vi "SequenceNodeUI.vi"() -> ()   [LabVIEW 2015, in "CleanupCategoryNode.lvclass"]
doc: "Copyright 2017 National Instruments Corporation\n\nLicensed under the Apache License, Version 2.0 (the \"License\"); you may not use this file except in compliance with the License. You may obtain a copy of the License at http://www.apache.org/licenses/LICENSE-2.0\nUnless required by applicable law or agreed to in writing, software distributed under the License is distributed on an \"AS IS\" BASIS, WITHOUT WARRANTIES OR CONDITIONS OF ANY KIND, either express or implied. See the License for the specific language governing permissions and limitations under the License."
uses:
  CleanupCategoryNode.lvclass
  <vilib>/NI/Configuration Framework/Node/NodeRef.ctl
  <vilib>/NI/Configuration Framework/Node/NISE_CEF_Node.lvclass
  <vilib>/NI/AMC/Message Queue.ctl
  <vilib>/NI/AMC/Message.ctl
  <vilib>/NI/Tools/Keyed Array/KeyedArray.ctl
  <vilib>/NI/Configuration Framework/Node/UserEventRef.ctl
  <vilib>/NI/Configuration Framework/Controls/EventCluster.ctl
  <vilib>/NI/AMC/Create Single Message.vi
  <vilib>/NI/AMC/Update Message Routing Info.vi
  <vilib>/NI/AMC/Send Message.vi
  <vilib>/NI/AMC/AMC.lvlib
  <vilib>/NI/Tools/Keyed Array/Tools_KeyedArray.lvlib
  <vilib>/NI/Configuration Framework/NISE_CEF_TreeControl.lvlib
panel:
  in  "user event":T1
  in  "main queue":T2
  out "Category Name":string
  in  "node ref":T3
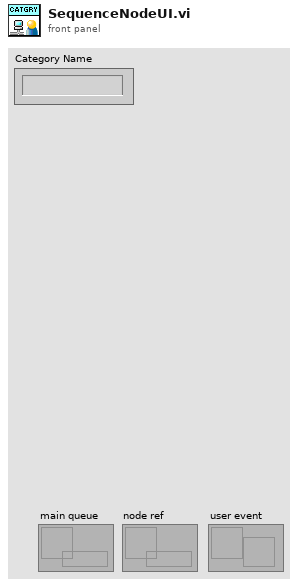
[diagram p1: front panel]
types:
  T1 = typedef "NISE_CEF_Node.lvclass/UserEventRef.ctl" = refnum<user-event>
  T2 = typedef "AMC.lvlib/Message Queue.ctl" = refnum<queue>
  T3 = typedef "NISE_CEF_Node.lvclass/NodeRef.ctl" = refnum<data-value>
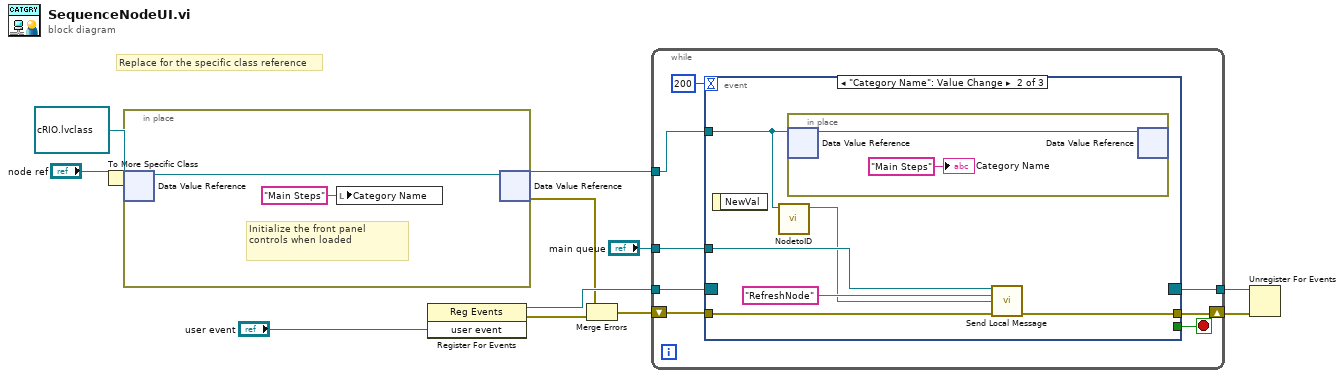
[diagram p0: block diagram]
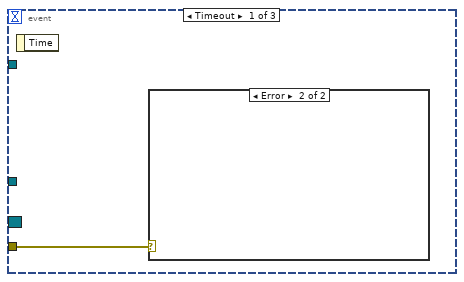
[diagram p2: hidden frame]
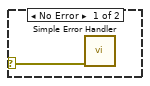
[diagram p3: hidden frame]
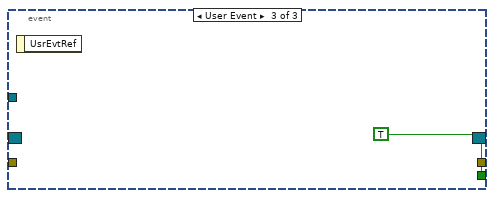
[diagram p4: hidden frame]
diagram:
  # "Replace for the specific class reference"
  n1 = To More Specific Class(target class=refnum<data-value> refnum ("data value reference"), reference="node ref") -> (specific class reference=w5:refnum<data-value>)  [unwired: 1 in, 1 out]
  n2 = in-place {
    # "Initialize the front panel controls when loaded"
    n3 = in-place-dvr #1(w5) -> (w14:refnum<class "CleanupCategoryNode.lvclass">)  [unwired: 1 out]
    n4 = local write "Category Name"("Main Steps" ("Category Name")) -> ()
    n5 = in-place-dvr #1(w14) -> (w12:refnum<data-value>, w2:errorcluster)
  }
  n6 = register-events("user event") -> (reference out=w9:refnum<event-registration>, error out=w3:errorcluster)  [unwired: 2 in]
  n7 = Merge Errors(w2, w3) -> (w1:errorcluster)
  n8 = while {
    tunnel: w12 -> [w22]
    tunnel: "main queue" -> [w21]
    tunnel: w9 -> [w19]
    tunnel: [w18] -> w8
    shift-right: [w16] -> w7
    shift-left: w1 -> [w15]
    stop <- w17 stop-if-true
    n9 = event shown="[1] \"Category Name\": Value Change" {
      selector: w19 -> [_ _ _]
      dyn-events: [_ _ _] -> w18
      timeout: 200 -> [_ _ _]
      tunnel: w22 -> [_ w28 _]
      tunnel: w21 -> [_ w29 _]
      tunnel: [_ _ TRUE] -> w17
      tunnel: [_ w26 _] -> w16
      tunnel: w15 -> [w23 w25 _]
      event Timeout {
        n10 = event-data() -> ()  [unwired: 1 in, 1 out]
        n11 = case shown="Error" w23 {
          selector: w23 -> [w24 _]
          frame No Error {
            n12 = call <vilib>:"Simple Error Handler.vi"("error in (no error)"=w24) -> ()  [unwired: 4 in, 5 out]
          }
          frame Error {
          }
        }
      }
      event "Category Name": Value Change {
        n13 = event-data() -> ()  [unwired: 1 in, 1 out]
        n14 = call <vilib>:"NodetoID.vi"("node ref"=w28) -> ("ID"=w27:string)  [unwired: 9 in, 1 out]
        n15 = in-place {
          n16 = in-place-dvr #2(w28) -> (w32:refnum<class "CleanupCategoryNode.lvclass">)  [unwired: 1 out]
          n17 = in-place-dvr #2(w32) -> ()  [unwired: 2 out]
          "Category Name" <- "Main Steps" ("Category Name")
        }
        n18 = call <vilib>:"Send Local Message.vi"("message queue in"=w29, "message name"="RefreshNode" ("Message Name"), "message value"=w27, "error in"=w25) -> ("error out"=w26:errorcluster)  [unwired: 9 in, 2 out]
      }
      event User Event {
        n19 = event-data() -> ()  [unwired: 1 in, 1 out]
      }
    }
  }
  n20 = Unregister For Events(event registration refnum=w8, error in=w7) -> ()  [unwired: 1 out]
